vi "Double.vi"(8 "Error In":errorcluster, 11 "number in":i32) -> (0 "Error Out":errorcluster, 3 "number out":i32)   [LabVIEW 2014]
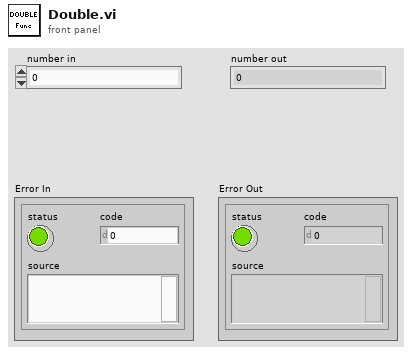
[diagram p1: front panel]
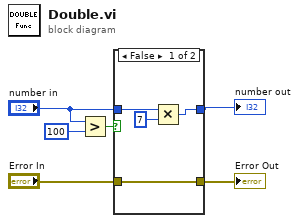
[diagram p0: block diagram]
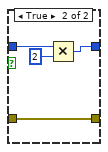
[diagram p2: hidden frame]
diagram:
  n1 = Greater?(x="number in", y=100) -> (0:w3:bool)
  n2 = case shown="False" w3 {
    tunnel: "number in" -> [w10 w14]
    tunnel: [w9 w13] -> w6
    tunnel: [w7 w11] -> w5
    tunnel: "Error In" -> [w7 w11]
    frame False {
      n3 = Multiply(x=w10, y=7) -> (x*y=w9:i32)
    }
    frame True {
      n4 = Multiply(x=w14, y=2) -> (x*y=w13:i32)
    }
  }
  "Error Out" <- w5
  "number out" <- w6
